vi "schleife temp.vi"() -> ()   [LabVIEW 2010]
panel:
  out "*(type *) &x 2":i32
  out "*(type *) &x":i32
  out "Anzahl der Zustände":i32
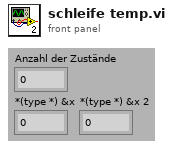
[diagram p1: front panel]
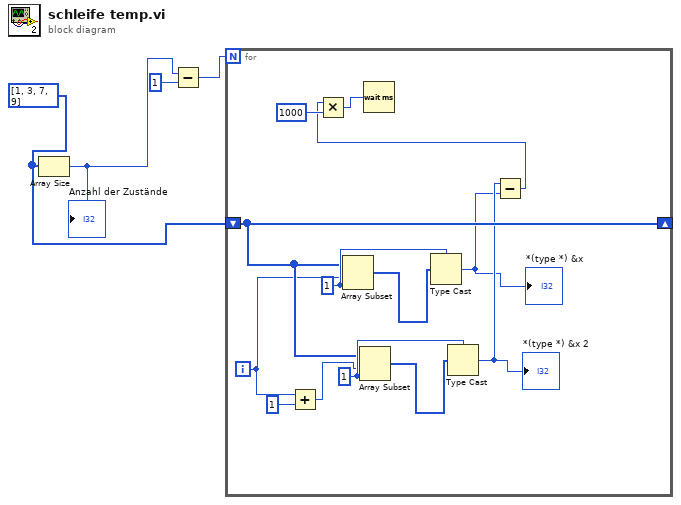
[diagram p0: block diagram]
diagram:
  w4 = i32[] [1, 3, 7, 9]
  n1 = Array Size(array=w4) -> (size(s)=w3:i32)
  "Anzahl der Zustände" <- w3
  n2 = Subtract(x=w3, y=1) -> (x-y=w1:i32)
  n3 = for {
    N: w1 -> [_]
    shift-right: [w11] -> _
    shift-left: w4 -> [w11]
    i -> [w10]
    w13 = 1 ("Länge")
    w16 = 1 ("Länge")
    n4 = Add(x=w10, y=1) -> (x+y=w8:i32)
    n5 = Array Subset(array=w11, index=w10, length=w16) -> (w15:i32[])
    n6 = Array Subset(array=w11, index=w8, length=w13) -> (w12:i32[])
    n7 = Type Cast(type=w16, x=w15) -> (*(type *) &x=w6:i32)
    "*(type *) &x" <- w6
    n8 = Type Cast(type=w13, x=w12) -> (*(type *) &x=w7:i32)
    "*(type *) &x 2" <- w7
    n9 = Subtract(x=w7, y=w6) -> (x-y=w5:i32)
    n10 = Multiply(x=w5, y=1000) -> (x*y=w14:i32)
    n11 = Wait (ms)(milliseconds to wait=w14) -> ()  [unwired: 1 out]
  }
